vi "3.7-Any_UDP_Server.vi"(3 "Multicast Address":u32, 4 "error In":errorcluster, 5 "Data in":variant, 6 "Connection ID":refnum<k16>, 7 "Send To Port":u16=58432) -> (0 "warning out":errorcluster, 1 "Processed":string, 2 "Connection ID out":refnum<k16>)   [LabVIEW 2010]
doc: "UDP Mutlicast Addressing Scheme:\n\n3.7 - Multicast Address: 133.7.3.7\n3.1-4.7.1 Port: 31471\n3.2-4.7.2 Port: 32472\n3.3-4.7.3 Port: 33473\n3.4-4.7.4 Port: 34474\n\n5.7 - Multicast Address: 133.7.5.7\n5.1-4.7.1 Port: 51471\n5.2-4.7.2 Port: 52472\n5.3-4.7.3 Port: 53473\n5.4-4.7.4 Port: 54474\n\n5.1-6.7.1 Port: 51671\n5.2-6.7.2 Port: 52672\n5.3-6.7.3 Port: 53673\n5.4-6.7.4 Port: 54674\n\n7.7 - Multicast Address: 133.7.7.7\n7.1-6.7.1 Port: 61671\n7.2-6.7.2 Port: 62672\n7.3-6.7.3 Port: 63673\n7.4-6.7.4 Port: 64674"
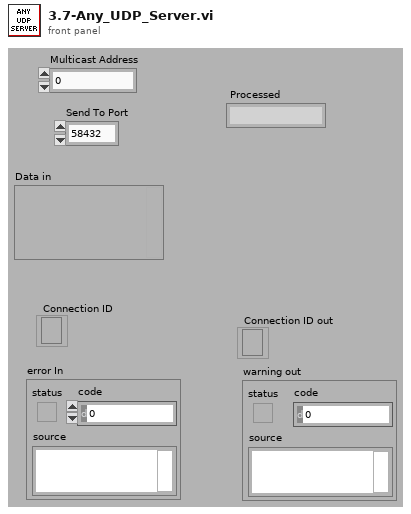
[diagram p1: front panel]
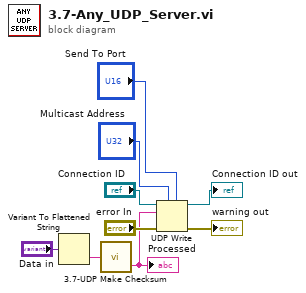
[diagram p0: block diagram]
diagram:
  n1 = Variant To Flattened String(Variant="Data in") -> (data string=w4:string)  [unwired: 1 out]
  n2 = call "3.7-UDP Make Checksum.vi"("Data String In"=w4) -> ("CS String Out"=w3:string)  [unwired: 1 out]
  "Processed" <- w3
  n3 = UDP Write(address="Multicast Address", port or service name="Send To Port", connection ID="Connection ID", data in=w3, 8:"error In") -> (error out=→"warning out":errorcluster, 3:→"Connection ID out":refnum<k16>)  [unwired: 1 in]
